vi "Drive Controller.vi"(8 "error in":errorcluster) -> ()   [LabVIEW 2016]
doc: "This VI executes continuously carrying out the current operation and responding to updates or new operation requests. It will often contain the timing or control code that is difficult to place directly in TeleOp. This VI generally opens all sensors and motors and isolates the rest of the robot code from knowing implementation details of how the operations are carried out."
uses:
  Drive Setpoints.ctl
  Drive Operations.ctl
  <vilib>/Rock Robotics/WPI/SafetyOutput/WPI_SafetyOutputConfigMenu.ctl
  <vilib>/Rock Robotics/SystemInterfaces/DIO/FPGA_DIOPWMChannel.ctl
  <vilib>/Rock Robotics/WPI/RobotDrive/WPI_RobotDriveOpen4MotorWithVictorSP.vi
  <vilib>/Rock Robotics/WPI/RobotDrive/WPI_RobotDriveMecanumDrive_Cartesian.vi
panel:
  out "Setpoints":T1(graph)
  out "Current\nCmd":string
  # "Tip: It may be helpful to observe inputs and sensor values.\nYou may also want to display tuning or debugging controls."
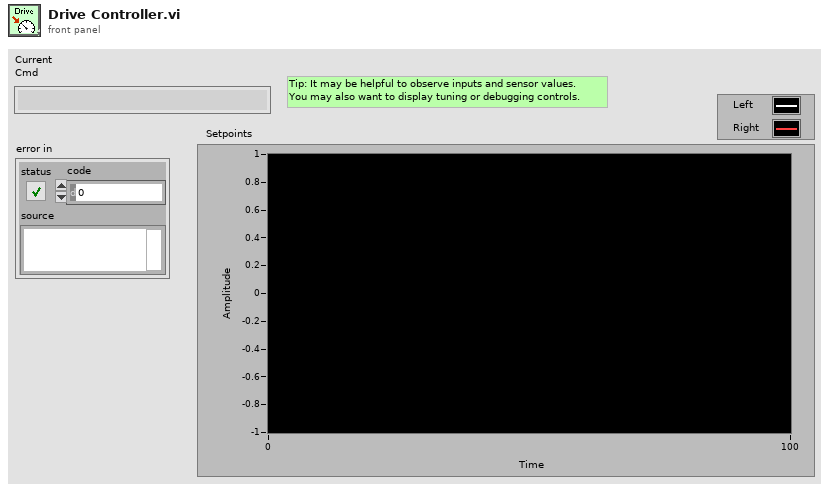
[diagram p1: front panel]
types:
  T1 = cluster{"Left Setpoint":dbl, "Right Setpoint":dbl}
  T2 = typedef "FPGA_DIOPWMChannel.ctl" = enum8{"PWM 0", "PWM 1", "PWM 2", "PWM 3", "PWM 4", "PWM 5", "PWM 6", "PWM 7", "PWM 8", "PWM 9", "PWM MXP 0", "PWM MXP 1", "PWM MXP 2", "PWM MXP 3", "PWM MXP 4", "PWM MXP 5", "PWM MXP 6", "PWM MXP 7", "PWM MXP 8", "PWM MXP 9", "Invalid"}
  T3 = typedef "WPI_SafetyOutputConfigMenu.ctl" = enum16{"Enable", "Disable"}
  T4 = typedef "Drive Setpoints.ctl" = cluster{"Operation":T5, "X Setpoint":dbl, "Y Setpoint":dbl, "Duration":dbl, "Twist Setpoint":dbl}
  T5 = typedef "Drive Operations.ctl" = enum16{"Reserve", "Read Current", "Immediate", "Drive for Time", "Drive for Distance"}
  T6 = typedef "WPI_RobotDriveDevRef.ctl" = cluster{"DevStatus":errorcluster, "Motors[]":T7[], "Square Inputs":bool, "Max Output":dbl}
  T7 = typedef "WPI_MotorControlDeviceRef.ctl" = cluster{"DeviceStatus":errorcluster, "Type":T8, "PWM":cluster{"PWM Channel":T2, "DeadBand":T9}, "CAN":cluster{"Device Number":u8, "SetOutput VI Ref":variant, "GetOutput VI Ref":variant, "Enable VI Ref":variant, "Disable VI Ref":variant, "Data":variant}, "Invert":bool}
  T8 = typedef "WPI_MotorControlType.ctl" = enum16{"PWM", "CAN"}
  T9 = typedef "WPI_PWMDeadband.ctl" = cluster{"Name":string, "maxPositivePwm":i32, "minPositivePwm":i32, "centerPwm":i32, "maxNegativePwm":i32, "minNegativePwm":i32, "angularRange":u16}
  T10 = typedef "Command Status Info.ctl" = cluster{"Name":string, "Status":T11, "notifier out":T12}
  T11 = typedef "Completion Status.ctl" = enum16{"Successful", "Aborted", "Incomplete"}
  T12 = typedef "Completion Notifier.ctl" = refnum<notifier>
  T13 = cluster{"SubSystem Data":T4, cluster{"Start Time (ms)":u32, "Iterations":i32}, cluster{"Command Info":T10, "Description":string, "SubSystem Data":T4, "notifier out":refnum<notifier>, "Subsystem Name":string}}
  T14 = cluster{"SubSystem Data":T4, cluster{"Start Time (ms)":u32, "Iterations":i32}, "Default Command Arguments":cluster{"Command Info":T10, "Description":string, "SubSystem Data":T4, "notifier out":refnum<notifier>, "Subsystem Name":string}}
  T15 = cluster{"Don't move motors while reserved":dbl, "Don't move motors while reserved":dbl}
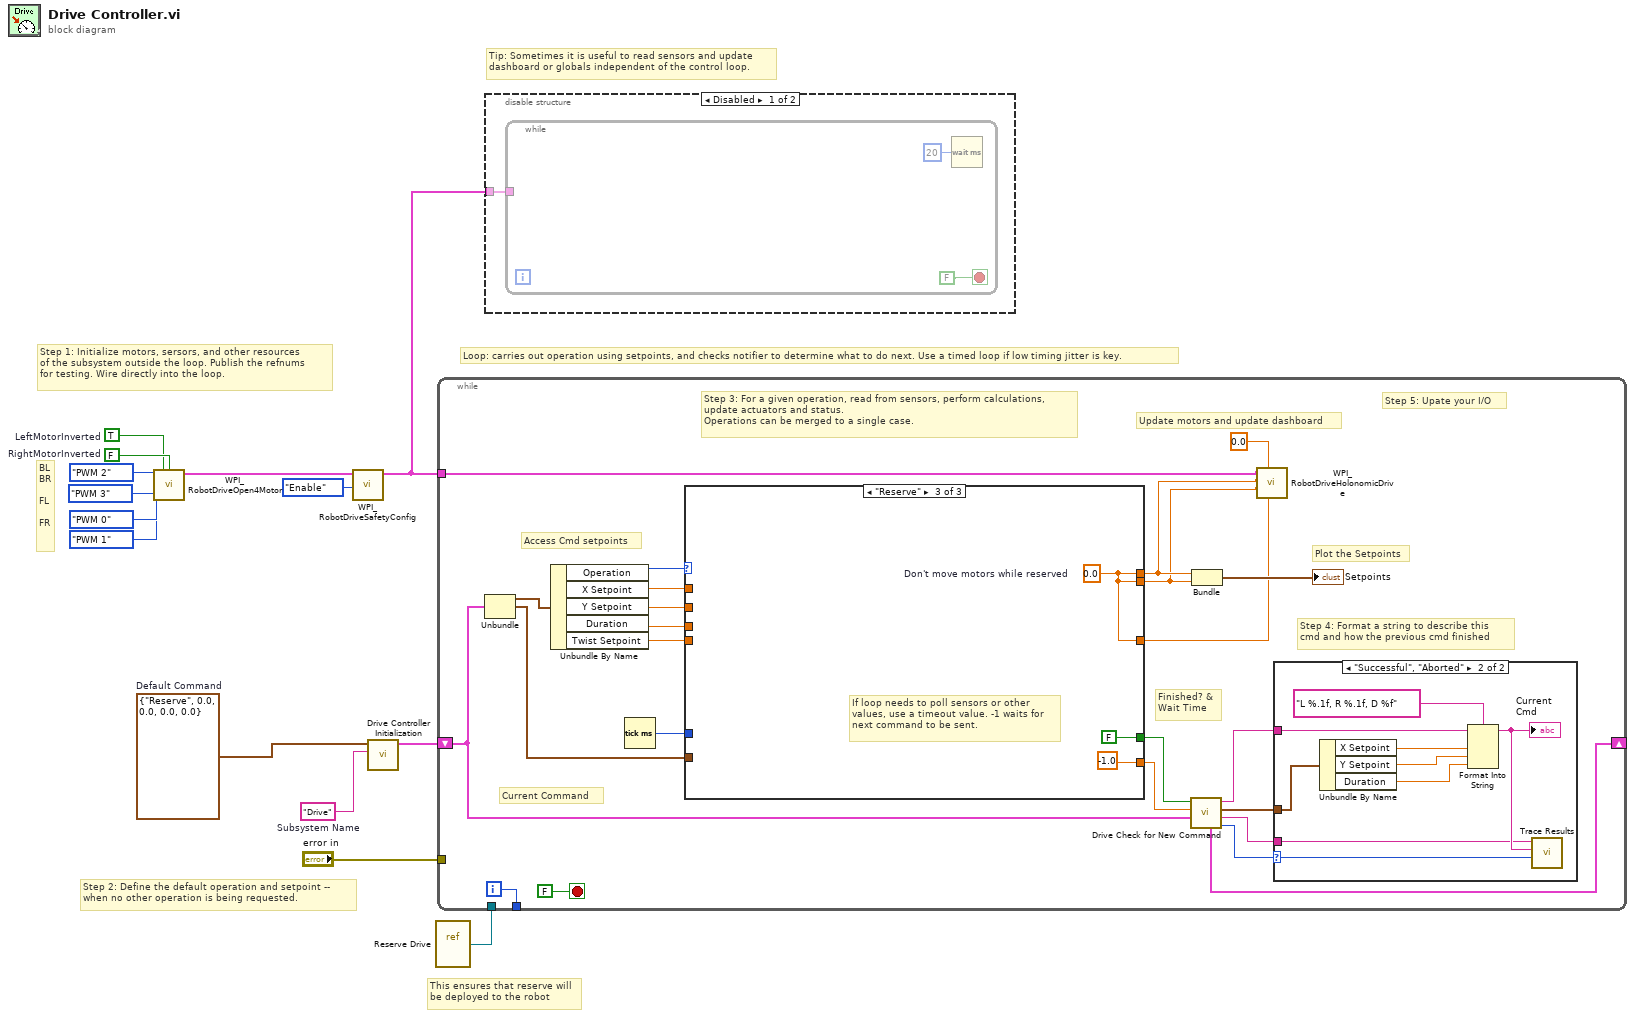
[diagram p0: block diagram]
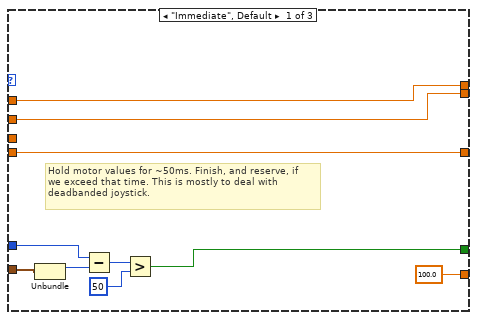
[diagram p4: hidden frame]
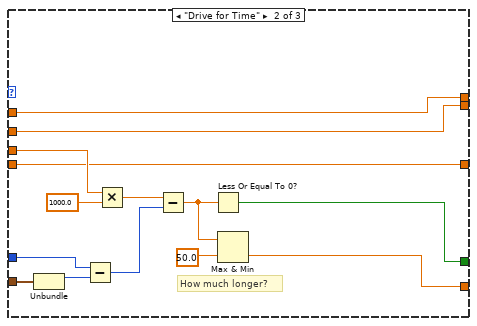
[diagram p5: hidden frame]
diagram:
  w11 = TRUE  # LeftMotorInverted
  w12 = FALSE  # RightMotorInverted
  w13 = T4 {"Operation"=enum."Reserve", "X Setpoint"=0.0, "Y Setpoint"=0.0, "Duration"=0.0, "Twist Setpoint"=0.0}  # Default Command
  w14 = "Drive"  # Subsystem Name
  # "BL\nBR\n\nFL\n\nFR"
  # "This ensures that reserve will\nbe deployed to the robot"
  # "Tip: Sometimes it is useful to read sensors and update\ndashboard or globals independent of the control loop."
  # "Step 2: Define the default operation and setpoint --\nwhen no other operation is being requested."
  # "Step 1: Initialize motors, sersors, and other resources\nof the subsystem outside the loop. Publish the refnums\nfor testing. Wire directly into the loop."
  # "Loop: carries out operation using setpoints, and checks notifier to determine what to do next. Use a timed loop if low timing jitter is key."
  n1 = call-poly <vilib>:"WPI_RobotDriveOpen4Motor.vi"("Rear Left Motor"=FPGA_DIOPWMChannel."PWM 2", "Rear Left Motor Inverted"=w11, "Rear Right Motor Inverted"=w12, "Rear Right Motor"=FPGA_DIOPWMChannel."PWM 3", "Front Left Motor"=FPGA_DIOPWMChannel."PWM 0", "Front Right Motor"=FPGA_DIOPWMChannel."PWM 1") -> ("RobotDriveDevRef"=w5:T6)  [unwired: 8 in, 1 out]
  n2 = call <vilib>:"WPI_RobotDriveSafetyConfig.vi"("mode"=WPI_SafetyOutputConfigMenu."Enable", "RobotDriveDevRef"=w5) -> ("RobotDriveDevRef"=w9:T6)  [unwired: 8 in, 1 out]
  n3 = call "Drive Controller Initialization.vi"("Subsystem Name"=w14, "Default Command"=w13) -> ("output cluster"=w7:T13)  [unwired: 9 in]
  n4 = vi-ref "Reserve Drive.vi"() -> (w6:refnum<vi>)
  n5 = while {
    shift-right: [w28] -> _
    shift-left: w7 -> [w21]
    tunnel: [w37] -> _
    tunnel: w9 -> [w19]
    tunnel: "error in" -> [_]
    tunnel: w6 -> [_]
    i -> [w37]
    stop <- FALSE stop-if-true
    # "Step 5: Upate your I/O"
    # "Step 4: Format a string to describe this\ncmd and how the previous cmd finished"
    # "Current Command"
    # "Update motors and update dashboard"
    # "Plot the Setpoints"
    # "Access Cmd setpoints"
    # "Finished? &\nWait Time"
    # "Step 3: For a given operation, read from sensors, perform calculations,\nupdate actuators and status.\nOperations can be merged to a single case."
    n6 = Unbundle(w21) -> ("SubSystem Data"=w35:T4, w22:cluster{"Start Time (ms)":u32, "Iterations":i32})  [unwired: 1 out]
    n7 = Unbundle By Name(w35) -> ("Operation"=w34:T5, "X Setpoint"=w33:dbl, "Y Setpoint"=w32:dbl, "Duration"=w31:dbl, "Twist Setpoint"=w20:dbl)
    n8 = Tick Count (ms)() -> (millisecond timer value=w30:u32)
    n9 = case shown="\"Reserve\"" w34 {
      tunnel: [100.0 w59 -1.0] -> w27
      tunnel: [w50 w66 FALSE ("ignore previous (F)")] -> w26
      tunnel: w22 -> [w49 w68 _]
      tunnel: [w56 w65 w72] -> w18
      tunnel: [w55 w64 w72] -> w17
      tunnel: w33 -> [w56 w65 _]
      tunnel: w32 -> [w55 w64 _]
      tunnel: w31 -> [_ w63 _]
      tunnel: w30 -> [w51 w62 _]
      tunnel: w20 -> [w48 w58 _]
      tunnel: [w48 w58 w72] -> w16
      frame "Immediate", Default {
        # "Hold motor values for ~50ms. Finish, and reserve, if\nwe exceed that time. This is mostly to deal with\ndeadbanded joystick."
        n10 = Unbundle(w49) -> ("Start Time (ms)"=w52:u32)  [unwired: 1 out]
        n11 = Subtract(x=w51, y=w52) -> (x-y=w53:u32)
        n12 = Greater?(x=w53, y=u8 50 ("Left Motor")) -> (0:w50:bool)
      }
      frame "Drive for Time" {
        # "How much longer?"
        n13 = Unbundle(w68) -> ("Start Time (ms)"=w67:u32)  [unwired: 1 out]
        n14 = Subtract(x=w62, y=w67) -> (x-y=w71:u32)
        n15 = Multiply(x=w63, y=1000.0) -> (x*y=w70:dbl)
        n16 = Subtract(x=w70, y=w71) -> (x-y=w61:dbl)
        n17 = Less Or Equal To 0?(x=w61) -> (x <= 0?=w66:bool)
        n18 = Max & Min(x=w61, y=50.0) -> (min(x,y)=w59:dbl)  [unwired: 1 out]
      }
      frame "Reserve" {
        w72 = 0.0  # Don't move motors while reserved
        # "If loop needs to poll sensors or other\nvalues, use a timeout value. -1 waits for\nnext command to be sent."
      }
    }
    n19 = call "Drive Check for New Command.vi"("input cluster"=w21, "Wait time (ms)"=w27, "Finished?"=w26) -> ("Completion"=w29:T11, "Subsystem Name"=w23:string, "SetPoint"=w24:T4, "Initial Trace String"=w25:string, "output cluster"=w28:T14)  [unwired: 4 in]
    n20 = Bundle("Don't move motors while reserved"=w18, "Don't move motors while reserved"=w17) -> (→"Setpoints":T15)  [unwired: 1 in]
    n21 = call-poly <vilib>:"WPI_RobotDriveHolonomicDrive.vi"("Rotation"=w16, "Gyro Angle"=0.0, "Y"=w17, "X"=w18, "RobotDriveDevRef"=w19) -> ()  [unwired: 4 in, 3 out]
    n22 = case shown="\"Successful\", \"Aborted\"" w29 {
      selector: w29 -> [_ w47]
      tunnel: w25 -> [_ w42]
      tunnel: w24 -> [_ w43]
      tunnel: w23 -> [_ w39]
      frame "Incomplete", Default {
        # "Continuing current command"
      }
      frame "Successful", "Aborted" {
        # "Report and setup for next command"
        n23 = Unbundle By Name(w43) -> ("X Setpoint"=w45:dbl, "Y Setpoint"=w46:dbl, "Duration"=w40:dbl)
        n24 = Format Into String(format string="L %.1f, R %.1f, D %f", initial string=w42, w45, w46, w40) -> (resulting string=w41:string)  [unwired: 1 in, 1 out]
        "Current\nCmd" <- w41
        n25 = call <vilib>:"Trace Results.vi"("Status of previous command"=w47, "Description"=w41, "Subsystem"=w39) -> ()  [unwired: 9 in]
      }
    }
  }
  n26 = disable-structure shown="Disabled" {
    disable-tunnel: w9 -> [w75 _]
    frame Disabled {
      n27 = while {
        tunnel: w75 -> [_]
        stop <- FALSE stop-if-true
        n28 = Wait (ms)(milliseconds to wait=u32 20) -> ()  [unwired: 1 out]
      }
    }
    frame Enabled {
    }
  }
